vi "Teardown.vi"(7 "Queue Actor in":refnum<class "Queue Actor.lvclass">, 11 "Teardown State in":refnum<class "Teardown State.lvclass">) -> (5 "Queue Actor out":refnum<class "Queue Actor.lvclass">)   [LabVIEW 2021, in "jettl.lvlib" / "Teardown State.lvclass"]
uses:
  Teardown State.lvclass
  Queue Actor/Queue Actor.lvclass
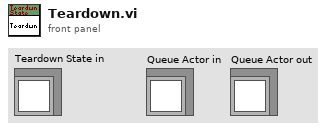
[diagram p1: front panel]
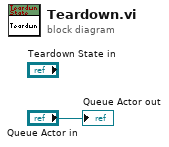
[diagram p0: block diagram]
diagram:
  "Queue Actor out" <- "Queue Actor in"
